vi "SVT SNR without Harmonics.vi"   [LabVIEW 2017, in "SoundVib_Distortion.lvlib"]
doc: "Performs a signal and noise analysis, including measuring the fundamental tone, and returns the detected fundamental frequency, detected fundamental amplitude, and signal-to-noise ratio (SNR) (without harmonics). The SNR measurement excludes harmonics of the fundamental frequency. Wire data to the <B>scaled signal [EU]</B> input to determine the polymorphic instance to use or manually select the instance.\n\nThe following formula calculates SNR:\n\nSNR = F / N\n\nwhere F is the fundamental tone RMS level and N is the noise RMS."
uses:
  <vilib>/addons/Sound and Vibration/svt_Distortion/SoundVib_Distortion.lvlib
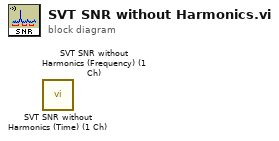
[diagram p0: block diagram]
diagram:
  n1 = call <vilib>:"SVT SNR without Harmonics (Time) (1 Ch).vi"() -> ()  [unwired: 12 in, 8 out]
  n2 = call <vilib>:"SVT SNR without Harmonics (Frequency) (1 Ch).vi"() -> ()  [unwired: 12 in, 8 out]
